vi "BorderHitStyle.vi"(10 "Border Hit Style":string) -> (2 "Used Border Hit Style":string)   [LabVIEW 2023]
uses:
  <vilib>/Utility/error.llb/whitespace.ctl
  <vilib>/Utility/error.llb/Trim Whitespace One-Sided.vi
panel:
  out "Possible Border Hit Styles":string[](array[string])
  in  "Default":string="o"
  out "Error":bool
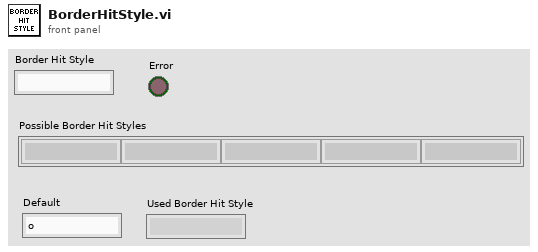
[diagram p1: front panel]
types:
  T1 = typedef "whitespace.ctl" = u16
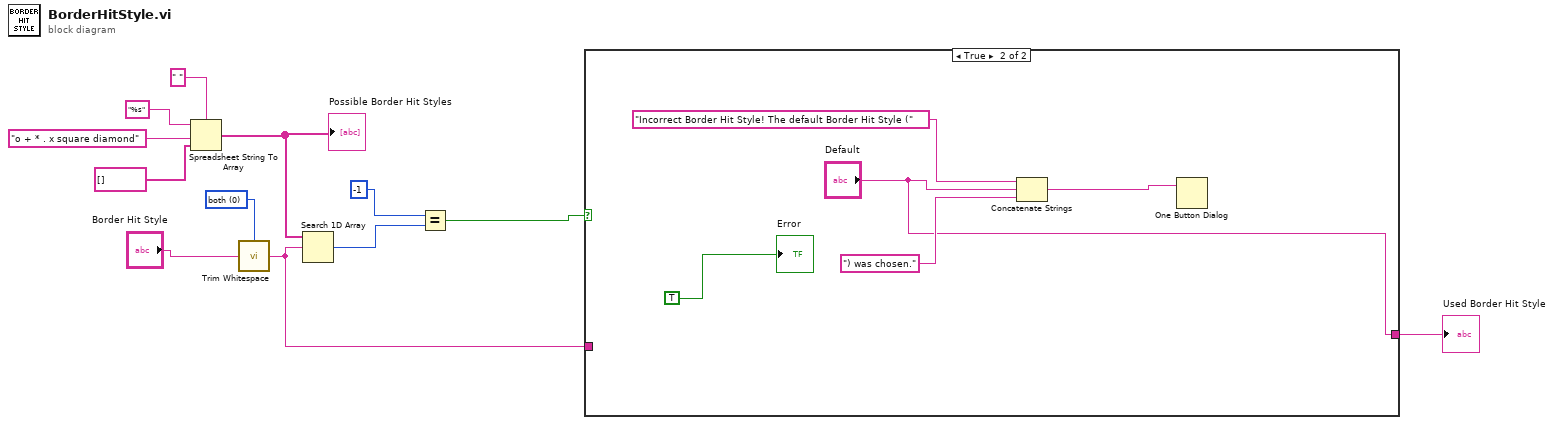
[diagram p0: block diagram]
diagram:
  w1 = T1 0 items=["both", "start of string", "end of string"] ("location (both)")
  n1 = Spreadsheet String To Array(delimiter (Tab)=" ", format string="%s", spreadsheet string="o + * . x square diamond", array type (2D Dbl)=string[] []) -> (array=w8:string[])
  "Possible Border Hit Styles" <- w8
  n2 = call <vilib>:"Trim Whitespace.vi"("string"="Border Hit Style", "location (both)"=w1) -> ("trimmed string"=w3:string)
  n3 = Search 1D Array(1D array=w8, element=w3) -> (index of element=w6:i32)  [unwired: 1 in]
  n4 = Equal?(x=-1, y=w6) -> (x = y?=w5:bool)
  n5 = case shown="True" w5 {
    tunnel: [w13 "Default"] -> w4
    tunnel: w3 -> [w13 _]
    frame False {
    }
    frame True {
      n6 = Concatenate Strings("Incorrect Border Hit Style! The default Border Hit Style (", "Default", ") was chosen.") -> (w14:string)
      n7 = One Button Dialog(message=w14) -> ()  [unwired: 1 in, 1 out]
      "Error" <- TRUE
    }
  }
  "Used Border Hit Style" <- w4
